vi "NewKickTo.vi"(0 "KickToSkill in":refnum<class "KickToSkill.lvclass">, 1 "Robot":refnum<class "Robot.lvclass">, 2 "State in":T1=enum."walk", 3 "use criteria?":bool, 4 "Game":refnum<class "Game.lvclass">, 5 "error in (no error)":errorcluster, 6 "firstCall?":bool=TRUE, 9 "Target":dbl[](array[numeric]), 13 "pass?":bool, 17 "chipKick ?":bool, 18 "ForceInGame":bool) -> (14 "KickToSkill out":refnum<class "KickToSkill.lvclass">, 15 "Robot out":refnum<class "Robot.lvclass">, 16 "State out":T1=enum."walk", 19 "error out":errorcluster)   [LabVIEW 2020, in "KickToSkill.lvclass"]
uses:
  KickToSkill.lvclass
  Robot_class/Robot.lvclass
  C:/Users/anton/Desktop/RoboIME/SSL_COMP/SSL_AI/Object_class/Object.lvclass
  Game_class/Game.lvclass
  Utilities_class/Utilities.lvclass
  Robot_class/robotKickToStates.ctl
  Robot_class/roles.ctl
  Team_class/OffensivePlay.ctl
  Robot_class/Robot.lvclass/Robot.ctl
  Game_class/Game.lvclass/Game.ctl
  Team_class/Team.lvclass/Team.ctl
  Object_class/Object.lvclass/Object.ctl
  Parameters_class/Parameters.lvclass/Parameters.ctl
  RobotFeedback/RobotFeedback.lvclass/RobotFeedback.ctl
  Robot_class/Write dest_x.vi
  Robot_class/Write dest_y.vi
  Robot_class/Write dest_orientation.vi
  Robot_class/Write dribble.vi
  RobotFeedback/Read dribblerContactToBall.vi
  <vilib>/Analysis/coordinate.llb/Wrap Angle (scalar).vi
  Robot_class/Read dest_orientation.vi
  Robot_class/Read orientation.vi
  Game_class/Read EnemyRef.vi
  Game_class/Read NewParameters.vi
  Game_class/Read FieldRef.vi
  Team_class/Read RobotRef.vi
  <vilib>/Analysis/_algsub.llb/Real Vector Norm.vi
  Object_class/Read x.vi
  Object_class/Read y.vi
  Robot_class/Write kick_x.vi
  Robot_class/Write kick_z.vi
  Parameters_class/Read ShootOutForce.vi
  Parameters_class/Read AttakingOurselves.vi
  Parameters_class/Read DistanceStop.vi
  Object_class/Read position(x,y).vi
  Game_class/Read BallRef.vi
  Game_class/Read Parameters.lvclass.vi
  Game_class/Read Utilities.lvclass.vi
  Game_class/Read OffensiveTeam.vi
  Game_class/Read Referee.vi
  Game_class/Read RobotsFeedback.vi
  Team_class/Read OffensivePlay.vi
  Parameters_class/Read timeoutToShoot.vi
  Parameters_class/Read ForceInGame.vi
  Parameters_class/Read Force++.vi
  Parameters_class/Read ChipKick activated.vi
  Parameters_class/Read KickEps.vi
  Parameters_class/Read KickRange.vi
  Parameters_class/Read MinDistToKick.vi
  Parameters_class/Read DistanceToKickingAngle.vi
  Parameters_class/Read KickAngle.vi
  Parameters_class/Read Enviroment.vi
  Parameters_class/Read KickForce.vi
  Parameters_class/Read TouchDistance.vi
  Parameters_class/Read Shoot Out_.vi
  Parameters_class/Read DistanceToConsiderRobotArrive.vi
  Robot_class/Read id.vi
  Robot_class/Write dest_x_kick.vi
  Robot_class/Write dest_y_kick.vi
  Robot_class/Read role.vi
  Robot_class/Write robotKickState.vi
  Enemy_class/Enemy.lvclass
  C:/Users/anton/Desktop/RoboIME/SSL_COMP/SSL_AI/Team_class/Team.lvclass
  Ally_class/Ally.lvclass
  Ball_class/Ball.lvclass
  Parameters_class/Read AttackerAngleToShootInDegrees.vi
  Parameters_class/Read AttackerAngleToTurnInDegrees.vi
  Field_class/Field.lvclass
  Parameters_class/Parameters.lvclass
  Referee_class/Referee.lvclass
  RobotFeedback/RobotFeedback.lvclass
  <vilib>/Analysis/NI_AAL_Angle.lvlib
  <vilib>/Analysis/NI_AALPro.lvlib
panel:
  out "difAngleRobotBall 4":dbl
  out "difAngleRobotBall 3":dbl
  out "firstCallArray":bool[](array[boolean])
  in  "AttackingOurselves":bool=TRUE
  out "?":refnum<class "Utilities.lvclass">
  out "difAngleRobotBall 2":dbl
  out "difAngleRobotBall":dbl
  out "difInDegrees":dbl
  out "orientationInDegrees":dbl
  out "?":refnum<class "Utilities.lvclass">
  out "?":refnum<class "Utilities.lvclass">
  in  "?":refnum<class "Utilities.lvclass">
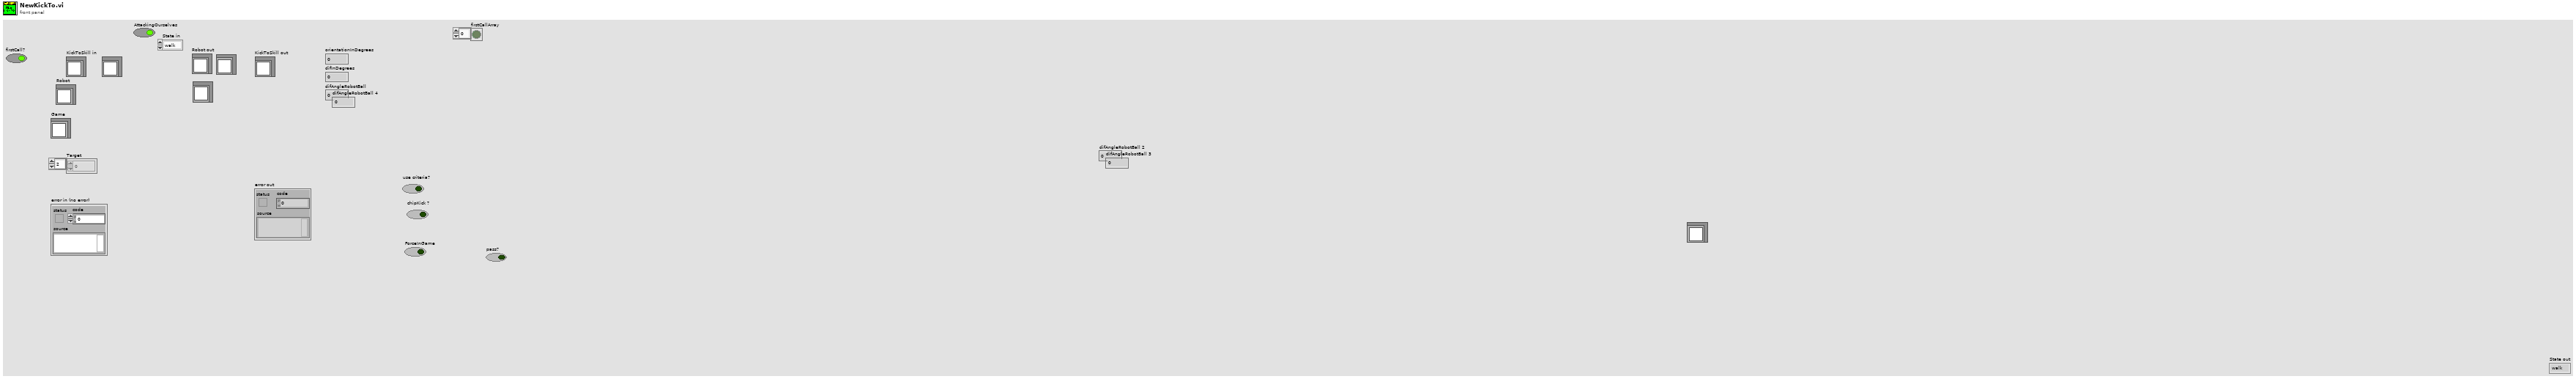
[diagram p1: front panel]
types:
  T1 = typedef "robotKickToStates.ctl" = enum16{"shootFromDirect", "avoidCollideBall", "goToBackBall", "none", "walk", "turn", "oldKickToShoot", "oldKickToGoToBackBall", "shoot"}
  T2 = typedef "OffensivePlay.ctl" = enum16{"5RobotsPassGamePlay", "5PreparePassGame", "5RobotsKeeperGame", "KeeperPassToStriker", "5RobotsNormalGamePlay", "PrepareKeeperPass", "ACBPass", "ABCPass", "PrepareTriplePass", "TableWithStriker", "TableWith2ndStrikerPlay", "PrepareDoublePass", "PrepareRollToPass", "SimplePass", "PreparePass", "PassToStriker", "BallOutOfField", "PassTo2ndStriker", "StopOffensive", "Prepare Penalty Enemy", "EnemyPossessionAtEnemyField", "EnemyPossesionAtOurField", "TestPlay", "PreparePenaltyAlly", "KickPenaltyAlly", "PrepareKickoffAlly", "PrepareKickoffEnemy", "IndirectEnemy", "DirectEnemy", "PreparePassInGame1", "NormalGame", "DirectKick", "Pass", "Halt", "Timeout", "PassPlay", "PenaltyEnemy"}
  T3 = typedef "roles.ctl" = enum16{"SimpleBallPlacement", "BallPlacementAllyPasser", "BallPlacementAllyReceiver", "BallPlacementEnemy", "5Robots5th", "PassBestReceiver", "5Robots4th", "5Robots3rd", "5Robots2nd", "5Robots1st", "PassBestRobot", "WaitPass", "ABCThirdKicker", "ABCFirstKicker", "ABCSecondKicker", "Tabler", "TableFinalizer", "PrepareRollToPassRoller", "PrepareRollToPassReceiver", "SimplePassRoll", "SimplePassRollReceiver", "PenaltyDefense", "PreparePassReceiver 2", "PreparePassReceiver 1", "PassObserver", "Timeout", "Goto", "ZigZag", "None", "BallOutOfField", "DefenderArea", "Duelist", "AttackerStop", "FollowAttacker", "KeeperRole", "KickPenalty", "AttackerAimGoal", "AttackerBlock", "Marker", "Halt", "Shoot", "PassKicker", "PassReceiver", "TestRole", "PenaltyAttacker"}
  T4 = typedef "NewParameters.ctl" = cluster{"PenaltyDistance":dbl, "DistanceAttackerToBackBall":dbl, "Division":enum16{"Div B", "Div A"}, "DistanceToAvoidyEnemyRobot":dbl, "BallPlacementDistance":dbl, "DisatanceBehindBallToStealBall":dbl, "MaxDistanceToPositionKickoff":dbl, "BlockEnemyTarget":bool, "MaxStopVAng":dbl, "DistanceMarkerToEnemy":dbl, "IgnoreDribblerContact":bool, "DistanceToBeginEnemyPosession":dbl, "GoToBallWhenEnemyNotMoving":bool, "EnemyDistanceToReduceVelocity":dbl, "TurnOnEnemyDistanceToReduceVelocity":bool, "EnemyDistanceToShootOutBall":dbl, "DefenseKickBall":bool, "MoreKickToGoal? (0-0.3)":dbl, "ChipKickInEnemyField":bool, "ShootOutRobotId":dbl, "FieldLenghtDenominatorInShootOut":dbl, "AdjustPositionInBallPlacement":bool, "PowerGodPass":dbl, "VelocityAbortEnemyPos":dbl, "MaxDistToBeginPass":dbl, "MinDistToBeginPass":dbl, "VelocityInDirects":dbl, "BadDribblerIDs":i32[], "NewKickToDistanceAroundBall":dbl, "PowerAvoidColisionMarker":dbl, "DistanceToAvoidColisionMarker":dbl, "AvoidBallKick":dbl, "DistanceTryKick":dbl, "SuicideKickDIstance":dbl, "FirstKickAtck":bool, "AdjustFirstKickDistance":dbl, "FirstKickDefense":bool, "AvoidAimLessKick":dbl, "DistanceToAvoidyEnemyShootRobot ":dbl, "NumberOfMarkers":dbl, "PotField":bool, "PIDLateral":bool, "MinDistanceFirstKickX":dbl, "MinDistanceFirstKickY":dbl, "FractionOfDistToTouchGround\nAfterChipKick":dbl, "FractionOfKickxWhen\nComposedWithKickz":dbl, "Style":T5, "MoveInTurnState":bool}
  T5 = typedef "Style.ctl" = enum16{"Insanity", "Offensive", "Defensive"}
  T6 = typedef "Enviroment.ctl" = enum16{"erForceSimulator", "grSim", "realGame"}
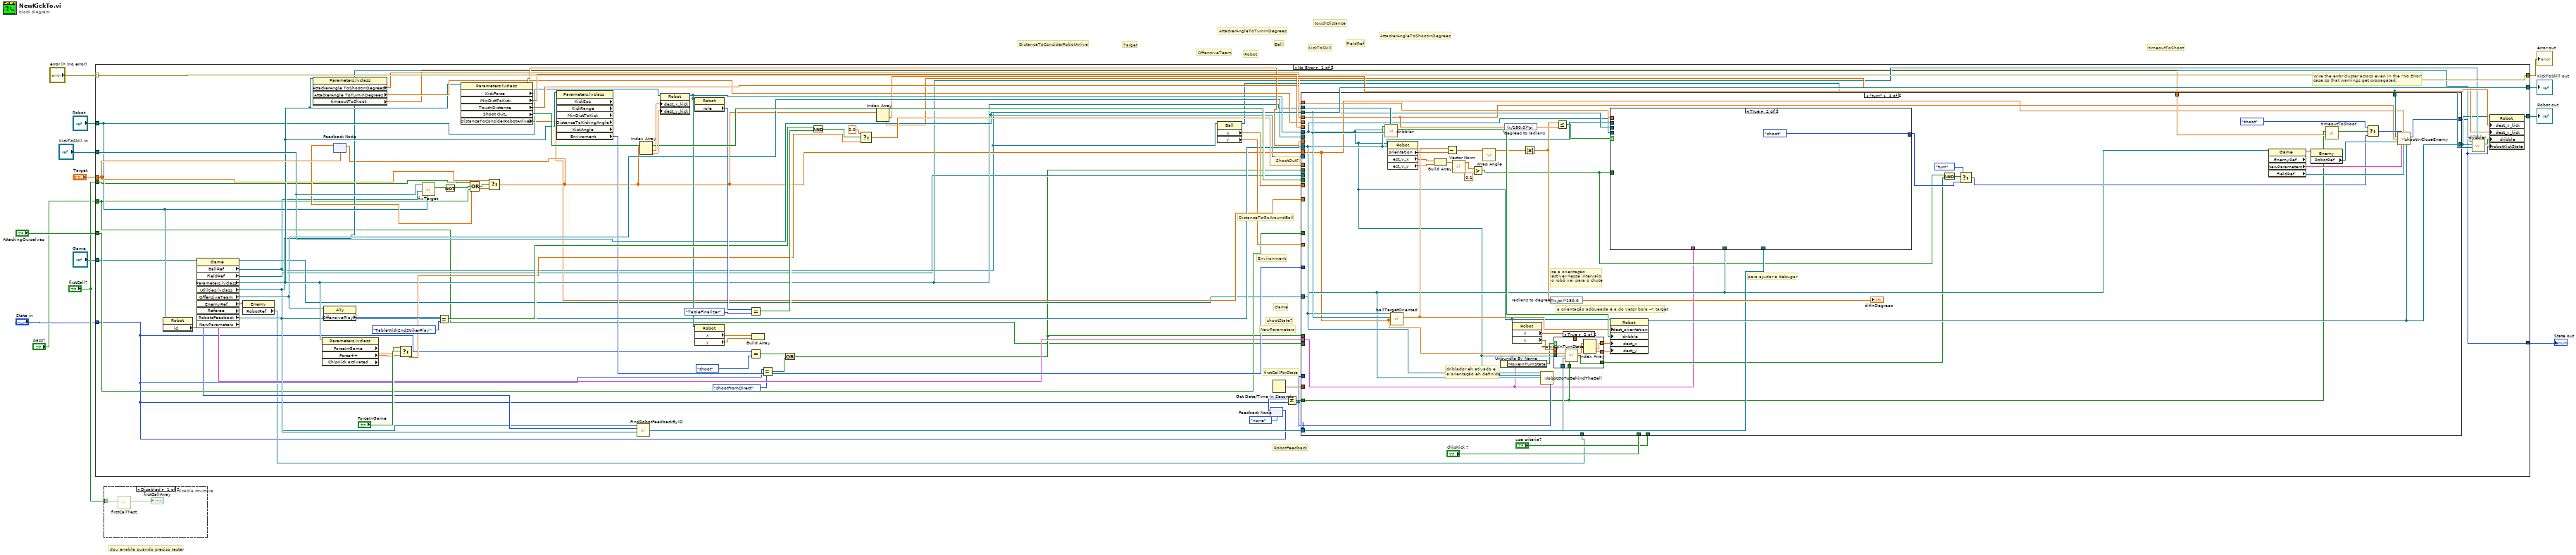
[diagram p0: block diagram]
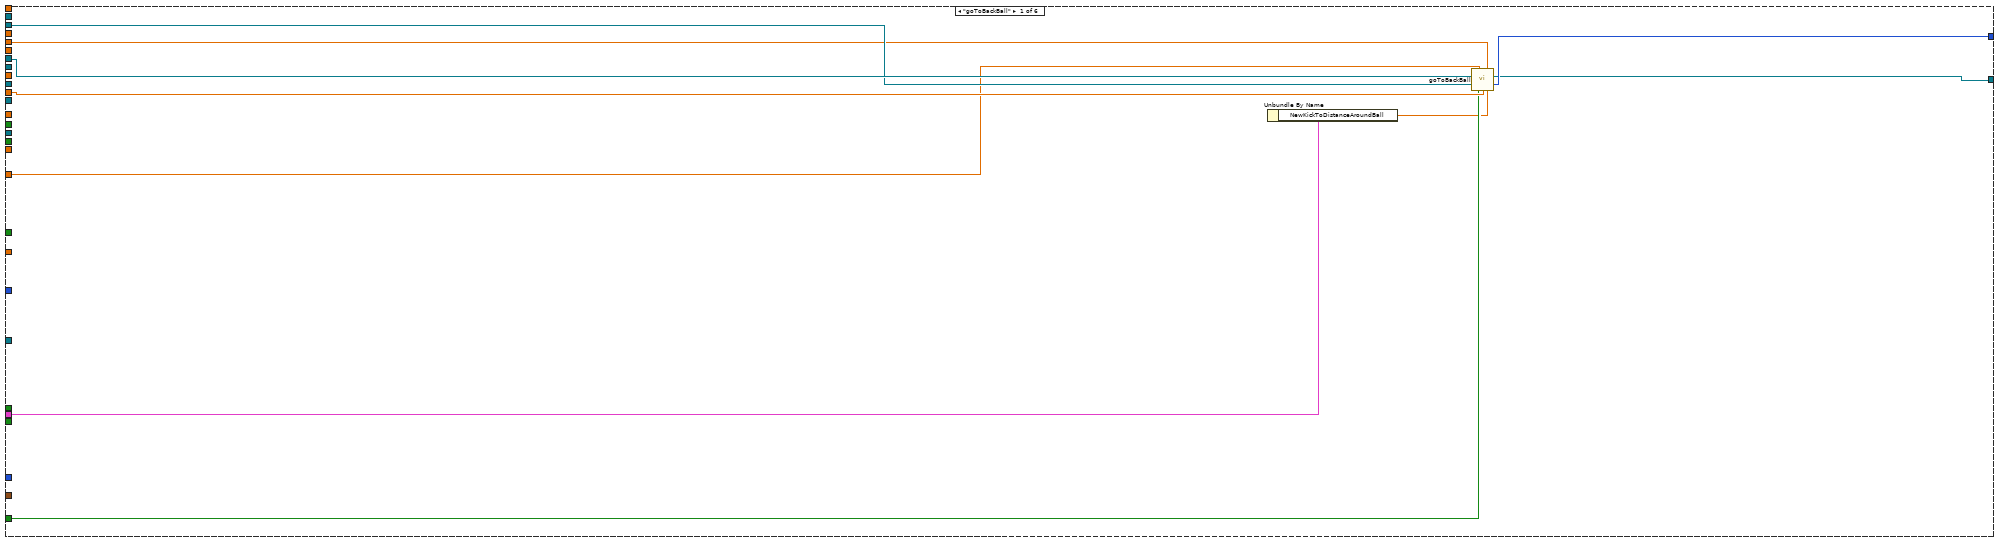
[diagram p2: hidden frame]
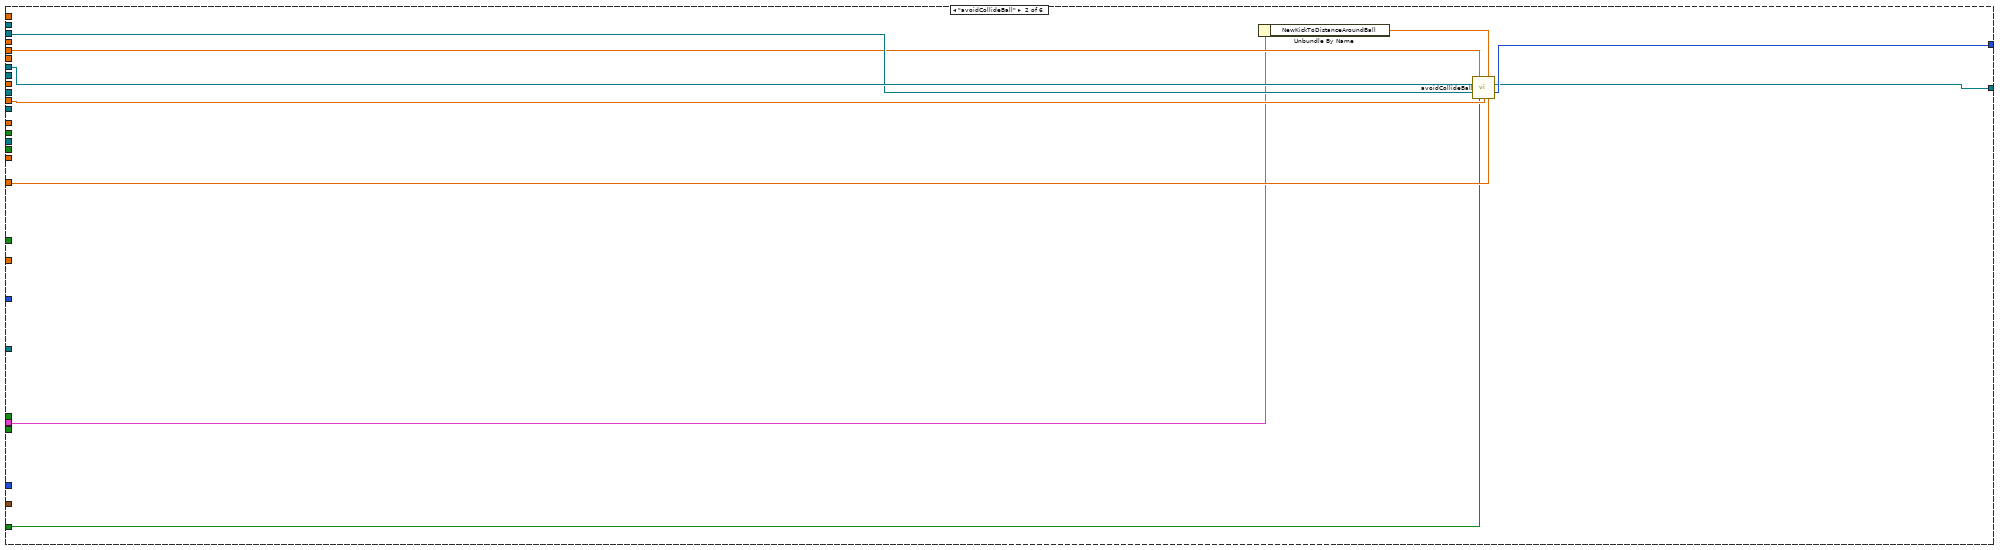
[diagram p3: hidden frame]
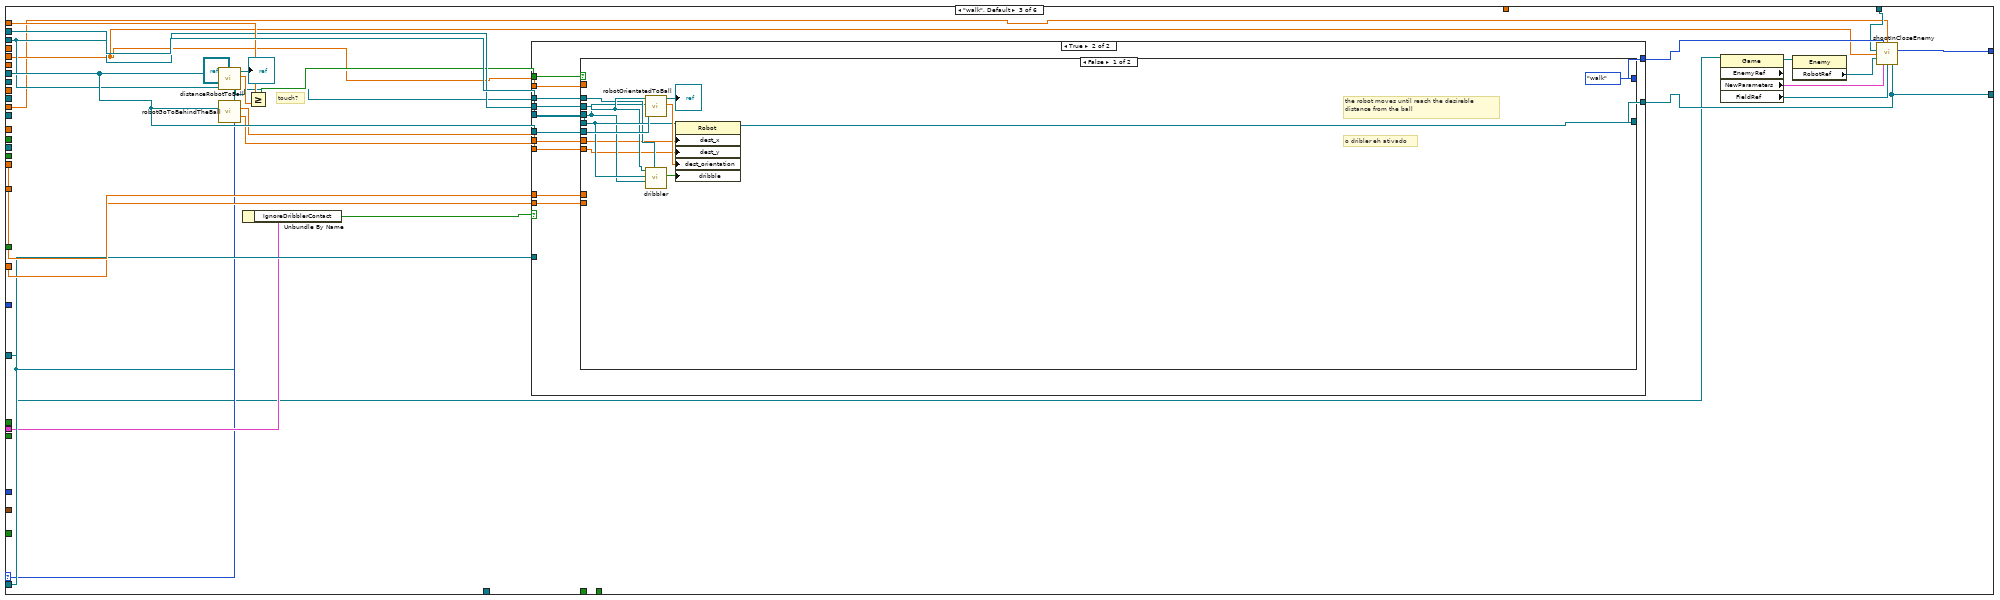
[diagram p4: hidden frame]
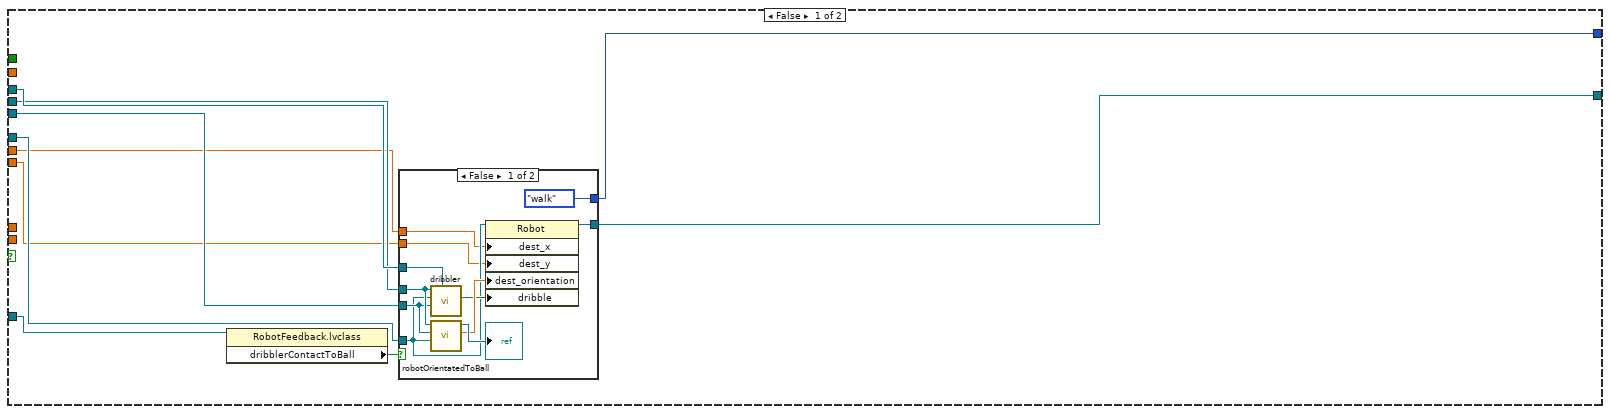
[diagram p5: hidden frame]
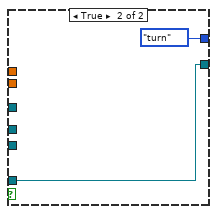
[diagram p6: hidden frame]
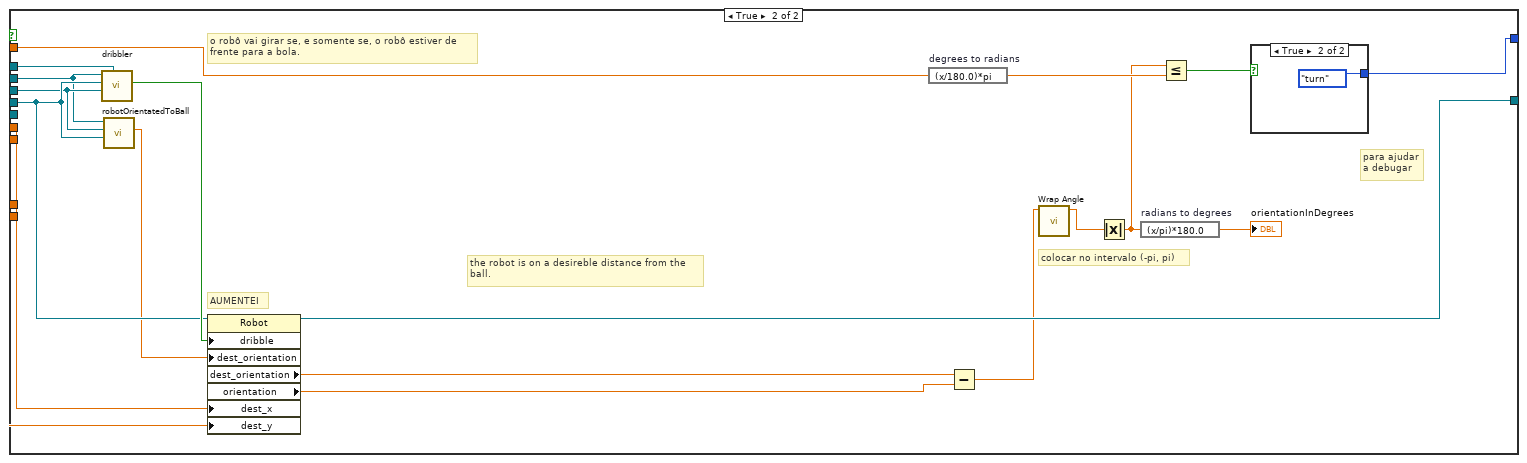
[diagram p7: hidden frame]
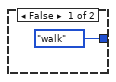
[diagram p8: hidden frame]
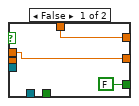
[diagram p9: hidden frame]
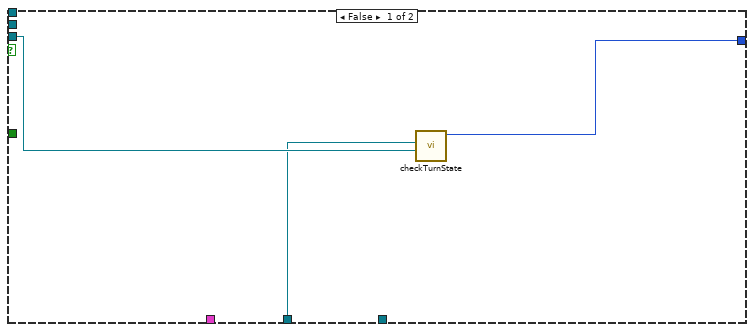
[diagram p10: hidden frame]
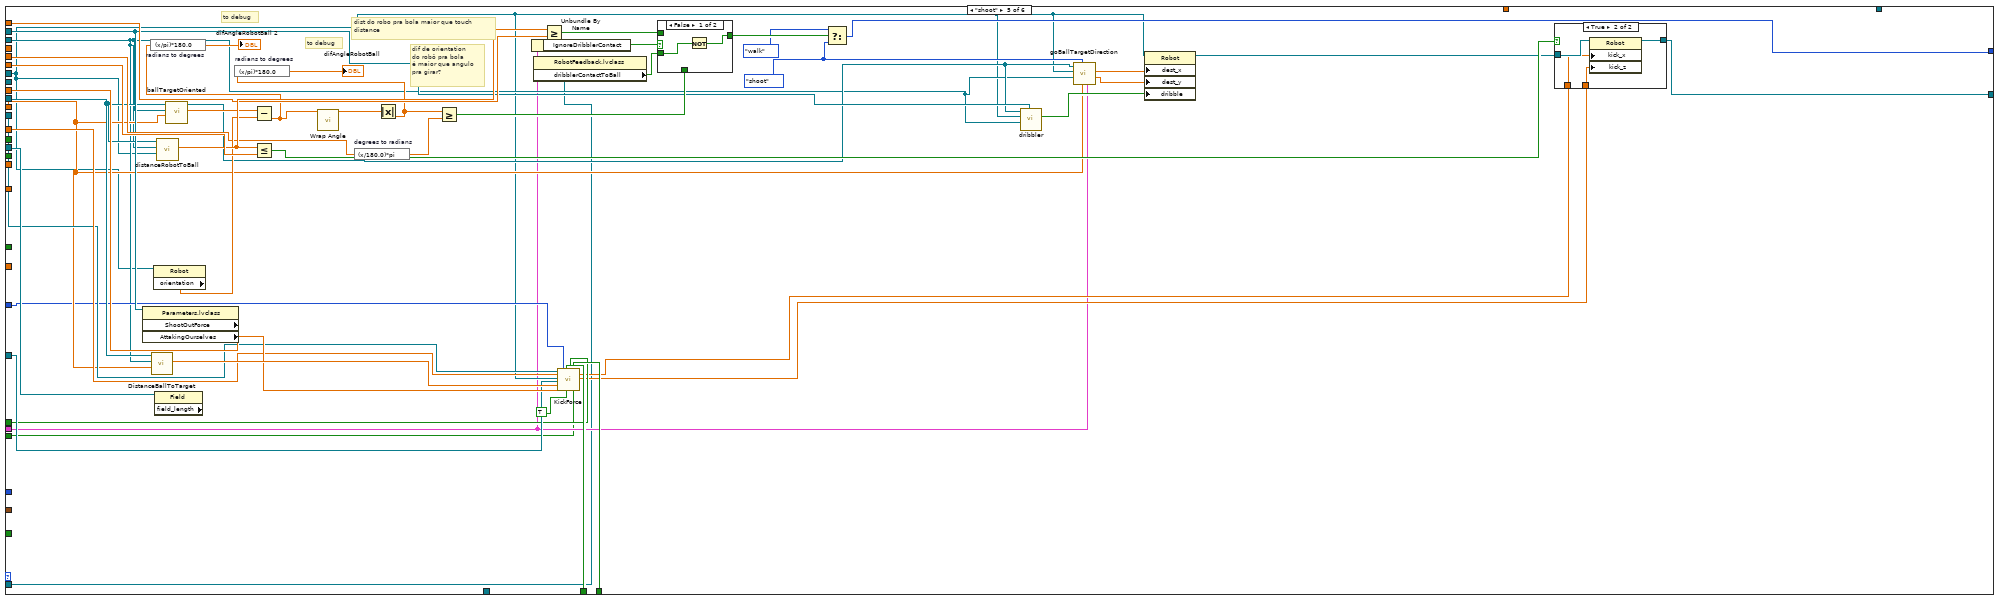
[diagram p11: hidden frame]
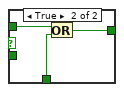
[diagram p12: hidden frame]
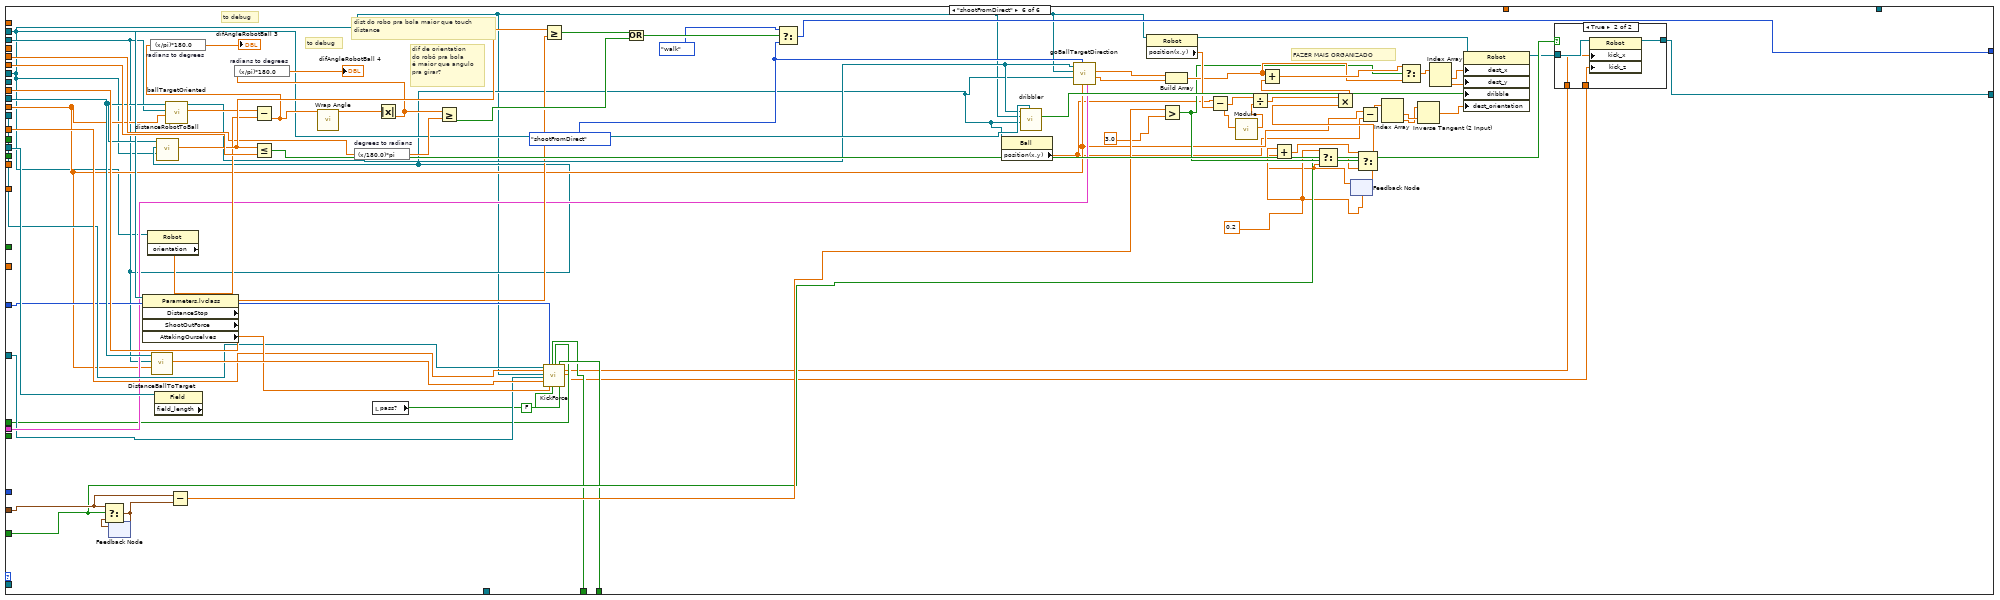
[diagram p14: hidden frame]
diagram:
  # "dou enable quando preciso testar"
  # "timeoutToShoot"
  # "AttackerAngleToShootInDegrees"
  # "touchDistance"
  # "AttackerAngleToTurnInDegrees"
  # "DistanceToConsiderRobotArrive"
  # "FieldRef"
  # "KickToSkill"
  # "Target"
  # "OffensiveTeam"
  # "Robot"
  # "Ball"
  n1 = case shown="No Error" "error in (no error)" {
    selector: "error in (no error)" -> [w86 w402]
    tunnel: [w86 w402] -> w12
    tunnel: [w61 w401] -> w10
    tunnel: "KickToSkill in" -> [w61 w401]
    tunnel: "Robot" -> [w49 w400]
    tunnel: [w57 w400] -> w8
    tunnel: "Game" -> [w27 _]
    tunnel: "Target" -> [w59 _]
    tunnel: "firstCall?" -> [w19 _]
    tunnel: "AttackingOurselves" -> [w43 _]
    tunnel: "State in" -> [w26 _]
    tunnel: [w25 _] -> w2
    tunnel: "pass?" -> [w16 _]
    frame No Error {
      # "RobotFeedback"
      # "shootState?"
      # "Game"
      # "NewParameters"
      # "firstCallForState"
      # "DistanceToGoAroundBall"
      # "Environment"
      # "ShootOut?"
      # "Wire the error cluster across even in the \"No Error\"\ncase so that warnings get propagated."
      n2 = property class="Robot"(reference=w49) -> ("id"=w48:i32)  [unwired: 1 in, 2 out]
      n3 = property class="Game" props=["BallRef", "FieldRef", "Parameters.lvclass", "Utilities.lvclass", "OffensiveTeam", "EnemyRef", "Referee", "RobotsFeedback", "NewParameters"](reference=w27) -> (reference out=w33:refnum<class "Game.lvclass">, "BallRef"=w32:refnum<class "Ball.lvclass">, "FieldRef"=w31:refnum<class "Field.lvclass">, "Parameters.lvclass"=w51:refnum<class "Parameters.lvclass">, "Utilities.lvclass"=w46:refnum<class "Utilities.lvclass">, "OffensiveTeam"=w60:refnum<class "Ally.lvclass">, "EnemyRef"=w15:refnum<class "Enemy.lvclass">, "RobotsFeedback"=w47:refnum<class "RobotFeedback.lvclass">[], "NewParameters"=w36:T4)  [unwired: 1 in, 2 out]
      n4 = property class="Enemy"(reference=w15) -> ("RobotRef"=w14:refnum<class "Robot.lvclass">[])  [unwired: 1 in, 2 out]
      n5 = property class="Parameters.lvclass"(reference=w51) -> ("AttackerAngle ToShootInDegrees"=w53:dbl, "AttackerAngle ToTurnInDegrees"=w54:dbl, "timeoutToShoot"=w37:dbl)  [unwired: 1 in, 2 out]
      n6 = property class="Parameters.lvclass" props=["ForceInGame", "Force++", "ChipKick activated"](reference=w51) -> ("ForceInGame"=w68:dbl, "Force++"=w67:dbl)  [unwired: 1 in, 3 out]
      n7 = property class="Ally"(reference=w60) -> ("OffensivePlay"=w73:T2)  [unwired: 1 in, 2 out]
      n8 = feedback #1(w59) -> (w58:dbl[])
      n9 = Select(t=w68, s="ForceInGame", f=w67) -> (s? t:f=w66:dbl)
      n10 = call "fixTarget.vi"("Robot"=w49, "Ball"=w32, "KickToSkill in"=w61) -> ("fixTarget?"=w24:bool)  [unwired: 6 in, 2 out]
      n11 = Equal?(x=w73, y=OffensivePlay."TableWith2ndStrikerPlay") -> (x = y?=w71:bool)
      n12 = Not(x=w24) -> (.not. x?=w18:bool)
      n13 = property class="Parameters.lvclass"(reference=w51) -> ("KickForce"=w78:dbl, "MinDistToKick"=w85:dbl, "TouchDistance"=w84:dbl, "Shoot Out_"=w79:bool, "DistanceToConsiderRobotArrive"=w41:dbl)  [unwired: 1 in, 2 out]
      n14 = Compound Arithmetic op=OR(w19, w18, w16) -> (w17:bool)
      n15 = Select(t=w59, s=w17, f=w58) -> (s? t:f=w42:dbl[])
      n16 = feedback-in #1(w42) -> ()
      n17 = property class="Parameters.lvclass" props=["KickEps", "KickRange", "MinDistToKick", "DistanceToKickingAngle", "KickAngle", "Enviroment"](reference=w51) -> ("Enviroment"=w45:T6)  [unwired: 1 in, 7 out]
      n18 = call "FindRobotFeedbackByID.vi"("RobotsFeedback"=w47, "id"=w48, "Utilities in"=w46) -> ("RobotFeedback.lvclass"=w44:refnum<class "RobotFeedback.lvclass">)  [unwired: 5 in, 3 out]
      n19 = Index Array(array=w42) -> (element #1=w81:dbl, element #2=w80:dbl)  [unwired: 2 in]
      n20 = property class="Robot"(reference=w49, "dest_x_kick"=w81, "dest_y_kick"=w80) -> (reference out=w62:refnum<class "Robot.lvclass">)  [unwired: 1 in, 1 out]
      n21 = property class="Robot"(reference=w62) -> ("role"=w76:T3)  [unwired: 1 in, 2 out]
      n22 = property class="Robot"(reference=w62) -> ("x"=w65:dbl, "y"=w64:dbl)  [unwired: 1 in, 2 out]
      n23 = Equal?(x=w76, y=roles."TableFinalizer") -> (x = y?=w74:bool)
      n24 = Equal?(x=w26, y=robotKickToStates."shoot" ("robotKickState")) -> (x = y?=w30:bool)
      n25 = Build Array(w65, w64) -> ()  [unwired: 1 out]
      n26 = Equal?(x=w26, y=robotKickToStates."shootFromDirect") -> (x = y?=w29:bool)
      n27 = Or(x=w30, y=w29) -> (x .or. y?=w20:bool)
      n28 = And(x=w71, y=w74) -> (x .and. y?=w70:bool)
      n29 = Select(t=0.0, s=w70, f=w66) -> (s? t:f=w63:dbl)
      n30 = Index Array(array=w42) -> (element #1=w56:dbl, element #2=w55:dbl)  [unwired: 2 in]
      n31 = property class="Ball"(reference=w32) -> (reference out=w34:refnum<class "Ball.lvclass">, "x"=w82:dbl, "y"=w83:dbl)  [unwired: 1 in, 1 out]
      n32 = feedback #2(robotKickToStates."none" ("state out")) -> (w40:T1)
      n33 = feedback-in #2(w26) -> ()
      n34 = Get Date/Time In Seconds() -> (seconds since 1Jan1904=w35:timestamp)
      n35 = Not Equal?(x=w40, y=w26) -> (x != y?=w39:bool)
      n36 = case shown="\"turn\"" w26 {
        selector: w26 -> [_ _ w109 w225 _ _]
        tunnel: [w96 w106 w119 w235 w295 w378] -> w25
        tunnel: w82 -> [_ _ w133 _ _ _]
        tunnel: w83 -> [_ _ w132 _ _ _]
        tunnel: w62 -> [w94 w104 w129 w222 w277 w330]
        tunnel: [w95 w105 w112 w229 w310 w392] -> w50
        tunnel: w32 -> [w93 w103 w128 w241 w279 w332]
        tunnel: w51 -> [_ _ w131 w250 w286 w369]
        tunnel: w84 -> [_ _ w130 w246 w302 _]
        tunnel: w46 -> [_ _ _ w240 w285 w368]
        tunnel: w85 -> [_ _ _ _ w312 w394]
        tunnel: w78 -> [_ _ _ _ w307 w389]
        tunnel: w61 -> [_ _ _ _ w305 w387]
        tunnel: w60 -> [_ _ _ _ _ _]
        tunnel: w31 -> [_ _ _ _ w308 w390]
        tunnel: w79 -> [_ _ _ _ _ _]
        tunnel: w42 -> [w92 w102 w108 w223 w284 w338]
        tunnel: w63 -> [_ _ _ _ w306 w388]
        tunnel: w20 -> [_ _ _ _ _ _]
        tunnel: w54 -> [w90 w100 w111 _ w293 w376]
        tunnel: w53 -> [_ _ _ w228 _ _]
        tunnel: w26 -> [_ _ _ _ _ _]
        tunnel: w45 -> [_ _ _ _ w281 w367]
        tunnel: w44 -> [_ _ w121 w226 w269 _]
        tunnel: w43 -> [_ _ _ _ _ _]
        tunnel: w41 -> [w91 w101 _ _ _ _]
        tunnel: w39 -> [w89 w99 _ w220 _ w343]
        tunnel: w37 -> [_ _ _ w237 _ _]
        tunnel: w36 -> [w88 w98 w120 w203 w270 w364]
        tunnel: w35 -> [_ _ _ _ _ w362]
        tunnel: w34 -> [_ _ w117 w234 _ _]
        tunnel: w33 -> [_ _ w107 w224 w278 w331]
        tunnel: "chipKick ?" -> [_ _ _ _ w276 w327]
        tunnel: "use criteria?" -> [_ _ _ _ w275 w329]
        tunnel: w20 -> [_ _ _ _ w274 w328]
        tunnel: w16 -> [_ _ _ _ w266 _]
        tunnel: w14 -> [_ _ _ w221 _ _]
        frame "goToBackBall" {
          n37 = Unbundle By Name(w88) -> ("NewKickToDistanceAroundBall"=w87:dbl)
          n38 = call "goToBackBall.vi"("DistanceToConsiderRobotArrive"=w91, "AttackerAngle\nToTurnInDegrees"=w90, "Robot in"=w94, "Ball"=w93, "firstCallForState"=w89, "target"=w92, "DistanceToGoAroundBall"=w87) -> ("Robot out"=w95:refnum<class "Robot.lvclass">, "robotKickState"=w96:T1)  [unwired: 5 in, 2 out]
        }
        frame "avoidCollideBall" {
          n39 = Unbundle By Name(w98) -> ("NewKickToDistanceAroundBall"=w97:dbl)
          n40 = call "avoidCollideBall.vi"("AttackerAngle\nToTurnInDegrees"=w100, "DistanceToGoAroundBall"=w97, "Robot"=w104, "Ball"=w103, "firstCallForState"=w99, "Target"=w102, "DistanceToConsiderRobotArrive"=w101) -> ("Robot out"=w105:refnum<class "Robot.lvclass">, "robotKickState"=w106:T1)  [unwired: 5 in, 2 out]
        }
        frame "walk", Default {
          # "touch?"
          n41 = call "distanceRobotToBall.vi"("Robot"=w129, "Ball"=w128, "Utilities in"="?") -> ("Distance Robot To Ball"=w127:dbl, "Utilities out"=→"?":refnum<class "Utilities.lvclass">)  [unwired: 6 in, 1 out]
          n42 = call "robotGoToBehindTheBall.vi"("Utilities in"="?", "Robot"=w129, "Game"=w107, "State in"=w109) -> ("dest_x"=w124:dbl, "dest_y"=w123:dbl)  [unwired: 8 in, 2 out]
          n43 = Unbundle By Name(w120) -> ("IgnoreDribblerContact"=w110:bool)
          n44 = Greater Or Equal?(x=w130, y=w127) -> (x >= y?=w126:bool)
          n45 = case shown="True" w110 {
            tunnel: [w137 w168] -> w118
            tunnel: w133 -> [_ w167]
            tunnel: w132 -> [_ w166]
            tunnel: [w138 w165] -> w112
            tunnel: w131 -> [w142 w164]
            tunnel: w129 -> [w140 w163]
            tunnel: w128 -> [w136 w162]
            tunnel: w111 -> [_ w161]
            tunnel: w126 -> [_ w160]
            tunnel: w124 -> [w135 w159]
            tunnel: w123 -> [w134 w158]
            tunnel: "?" -> [w141 w157]
            tunnel: w121 -> [w143 _]
            frame False {
              n46 = property class="RobotFeedback.lvclass"(reference=w143) -> ("dribblerContactToBall"=w139:bool)  [unwired: 1 in, 2 out]
              n47 = case shown="False" w139 {
                tunnel: w142 -> [w151 _]
                tunnel: w141 -> [w150 _]
                tunnel: w136 -> [w149 _]
                tunnel: w140 -> [w148 w156]
                tunnel: [w147 w156] -> w138
                tunnel: [robotKickToStates."walk" robotKickToStates."turn" ("robotKickState")] -> w137
                tunnel: w135 -> [w145 _]
                tunnel: w134 -> [w144 _]
                frame False {
                  n48 = call "dribbler.vi"("Parameters.lvclass"=w151, "Ball"=w149, "Robot"=w148, "Utilities in"=w150) -> ("Dribbler?"=w152:bool)  [unwired: 5 in, 2 out]
                  n49 = call "robotOrientatedToBall.vi"("Robot"=w148, "BallRef"=w149, "Utilities in"=w150) -> ("Orientation"=w153:dbl, "Utilities out"=→"?":refnum<class "Utilities.lvclass">)  [unwired: 6 in, 1 out]
                  n50 = property class="Robot"(reference=w148, "dest_x"=w145, "dest_y"=w144, "dest_orientation"=w153, "dribble"=w152) -> (reference out=w147:refnum<class "Robot.lvclass">)  [unwired: 1 in, 1 out]
                }
                frame True {
                }
              }
            }
            frame True {
              n51 = case shown="False" w160 {
                tunnel: [robotKickToStates."walk" w198] -> w168
                tunnel: w167 -> [_ _]
                tunnel: w166 -> [_ _]
                tunnel: w163 -> [w176 w195]
                tunnel: [w180 w197] -> w165
                tunnel: w163 -> [w179 _]
                tunnel: w162 -> [w173 w194]
                tunnel: w157 -> [w175 w193]
                tunnel: w164 -> [w174 w199]
                tunnel: w159 -> [w171 w183]
                tunnel: w158 -> [w170 w182]
                tunnel: w161 -> [_ w181]
                frame False {
                  # "o dribler eh ativado"
                  # "the robot moves until reach the desireble \ndistance from the ball"
                  n52 = call "robotOrientatedToBall.vi"("Robot"=w179, "BallRef"=w173, "Utilities in"=w175) -> ("Orientation"=w177:dbl, "Utilities out"=→"?":refnum<class "Utilities.lvclass">)  [unwired: 6 in, 1 out]
                  n53 = call "dribbler.vi"("Parameters.lvclass"=w174, "Ball"=w173, "Robot"=w176, "Utilities in"=w175) -> ("Dribbler?"=w172:bool)  [unwired: 5 in, 2 out]
                  n54 = property class="Robot"(reference=w176, "dest_x"=w171, "dest_y"=w170, "dest_orientation"=w177, "dribble"=w172) -> (reference out=w180:refnum<class "Robot.lvclass">)  [unwired: 1 in, 1 out]
                }
                frame True {
                  # "para ajudar\na debugar"
                  # "colocar no intervalo (-pi, pi)"
                  # "AUMENTEI"
                  # "o robô vai girar se, e somente se, o robô estiver de frente para a bola."
                  # "the robot is on a desireble distance from the\nball."
                  n55 = call "dribbler.vi"("Parameters.lvclass"=w199, "Ball"=w194, "Robot"=w195, "Utilities in"=w193) -> ("Dribbler?"=w196:bool)  [unwired: 5 in, 2 out]
                  n56 = call "robotOrientatedToBall.vi"("Robot"=w195, "BallRef"=w194, "Utilities in"=w193) -> ("Orientation"=w192:dbl)  [unwired: 6 in, 2 out]
                  n57 = property class="Robot"(reference=w195, "dribble"=w196, "dest_orientation"=w192, "dest_x"=w183, "dest_y"=w182) -> (reference out=w197:refnum<class "Robot.lvclass">, "dest_orientation"=w190:dbl, "orientation"=w189:dbl)  [unwired: 1 in, 1 out]
                  n58 = expression code="(x/180.0)*pi" "degrees to radians"(w181) -> (w191:dbl)
                  n59 = Subtract(x=w190, y=w189) -> (x-y=w187:dbl)
                  n60 = call-poly <vilib>:"Wrap Angle.vi"("angle in"=w187) -> ("angle out"=w186:dbl)  [unwired: 9 in, 1 out]
                  n61 = Absolute Value(x=w186) -> (abs(x)=w184:dbl)
                  n62 = expression code="(x/pi)*180.0" "radians to degrees"(w184) -> (→"orientationInDegrees":dbl)
                  n63 = Less Or Equal?(x=w184, y=w191) -> (x <= y?=w188:bool)
                  n64 = case shown="True" w188 {
                    tunnel: [robotKickToStates."walk" robotKickToStates."turn" ("robotKickState")] -> w198
                    frame False {
                    }
                    frame True {
                    }
                  }
                }
              }
            }
          }
          n65 = property class="Game"(reference=w107) -> ("EnemyRef"=w116:refnum<class "Enemy.lvclass">, "NewParameters"=w114:T4, "FieldRef"=w113:refnum<class "Field.lvclass">)  [unwired: 1 in, 2 out]
          n66 = property class="Enemy"(reference=w116) -> ("RobotRef"=w115:refnum<class "Robot.lvclass">[])  [unwired: 1 in, 2 out]
          n67 = call "shootInCloseEnemy.vi"("robotKickState In"=w118, "Target"=w108, "Ball"=w117, "AttackerAngle ToShootInDegrees"=w111, "EnemyRoboRef"=w115, "NewParameters"=w114, "FieldRef"=w113, "Robot in"=w112) -> ("robotKickState out"=w119:T1)  [unwired: 5 in, 2 out]
        }
        frame "turn" {
          # "para ajudar a debugar"
          # "a orientação adqueada é a do vetor bola -> target"
          # "se a orientação \nestiver nesse intervalo\no robô vai para o chute"
          # "driblador eh ativado e\na orientação eh definida"
          n68 = call "dribbler.vi"("Parameters.lvclass"=w250, "Ball"=w241, "Robot"=w222, "Utilities in"=w240) -> ("Dribbler?"=w247:bool)  [unwired: 5 in, 2 out]
          n69 = property class="Robot"(reference=w222) -> ("orientation"=w249:dbl, "est_v_x"=w216:dbl, "est_v_y"=w215:dbl)  [unwired: 1 in, 2 out]
          n70 = call "ballTargetOriented.vi"("Target"=w223, "Ball"=w241, "Utilities in"=w240) -> ("Orientation"=w239:dbl)  [unwired: 6 in, 2 out]
          n71 = Build Array(w216, w215) -> (w214:dbl[])
          n72 = Subtract(x=w239, y=w249) -> (x-y=w245:dbl)
          n73 = call-poly <vilib>:"Vector Norm.vi"("Input Vector"=w214) -> ("norm"=w213:dbl)  [unwired: 9 in, 1 out]
          n74 = Greater?(x=w213, y=0.1) -> (0:w207:bool)
          n75 = call-poly <vilib>:"Wrap Angle.vi"("angle in"=w245) -> ("angle out"=w244:dbl)  [unwired: 9 in, 1 out]
          n76 = Unbundle By Name(w203) -> ("MoveInTurnState"=w202:bool)
          n77 = expression code="(x/180.0)*pi" "degrees to radians"(w228) -> (w248:dbl)
          n78 = property class="Robot"(reference=w222) -> ("x"=w205:dbl, "y"=w204:dbl)  [unwired: 1 in, 2 out]
          n79 = Absolute Value(x=w244) -> (abs(x)=w243:dbl)
          n80 = call "robotGoToBehindTheBall.vi"("Utilities in"=w240, "Robot"=w222, "Game"=w224, "State in"=w225) -> ()  [unwired: 8 in, 4 out]
          n81 = expression code="(x/pi)*180.0" "radians to degrees"(w243) -> (→"difInDegrees":dbl)
          n82 = case shown="True" w202 {
            tunnel: w223 -> [_ w261]
            tunnel: w222 -> [_ w260]
            tunnel: w221 -> [_ w259]
            tunnel: w220 -> [_ w258]
            tunnel: [w253 w256] -> w219
            tunnel: [w252 w255] -> w218
            tunnel: [FALSE ("RobotToClose") w254] -> w208
            tunnel: w205 -> [w253 _]
            tunnel: w204 -> [w252 _]
            frame False {
            }
            frame True {
              n83 = call "movingInTurnState.vi"("Target"=w261, "Robot"=w260, "RobotRef"=w259, "first call"=w258) -> ("Dest"=w257:dbl[], "RobotToClose"=w254:bool)  [unwired: 8 in, 2 out]
              n84 = Index Array(array=w257) -> (element #1=w256:dbl, element #2=w255:dbl)  [unwired: 2 in]
            }
          }
          n85 = Less Or Equal?(x=w243, y=w248) -> (x <= y?=w217:bool)
          n86 = case shown="True" w217 {
            tunnel: [w262 robotKickToStates."shoot" ("robotKickState")] -> w210
            tunnel: w240 -> [_ _]
            tunnel: w222 -> [w264 _]
            tunnel: w241 -> [_ _]
            tunnel: w246 -> [_ _]
            tunnel: w203 -> [_ _]
            tunnel: w226 -> [_ _]
            tunnel: w224 -> [w263 _]
            tunnel: w207 -> [_ _]
            frame False {
              n87 = call "checkTurnState.vi"("Robot"=w264, "Game"=w263) -> ("robotKickState"=w262:T1)  [unwired: 9 in]
            }
            frame True {
            }
          }
          n88 = property class="Robot"(reference=w222, "dest_orientation"=w239, "dribble"=w247, "dest_x"=w219, "dest_y"=w218) -> (reference out=w229:refnum<class "Robot.lvclass">)  [unwired: 1 in, 1 out]
          n89 = And(x=w207, y=w208) -> (x .and. y?=w206:bool)
          n90 = Select(t=robotKickToStates."turn" ("robotKickState"), s=w206, f=w210) -> (s? t:f=w209:T1)
          n91 = property class="Game"(reference=w224) -> ("EnemyRef"=w233:refnum<class "Enemy.lvclass">, "NewParameters"=w231:T4, "FieldRef"=w230:refnum<class "Field.lvclass">)  [unwired: 1 in, 2 out]
          n92 = property class="Enemy"(reference=w233) -> ("RobotRef"=w232:refnum<class "Robot.lvclass">[])  [unwired: 1 in, 2 out]
          n93 = call "timeoutToShoot.vi"("timeoutToShoot"=w237, "firstCallForState"=w220) -> ("elapsedTimeToShoot"=w238:bool)  [unwired: 7 in, 2 out]
          n94 = Select(t=robotKickToStates."shoot" ("robotKickState"), s=w238, f=w209) -> (s? t:f=w236:T1)
          n95 = call "shootInCloseEnemy.vi"("robotKickState In"=w236, "Target"=w223, "Ball"=w234, "AttackerAngle ToShootInDegrees"=w228, "EnemyRoboRef"=w232, "NewParameters"=w231, "FieldRef"=w230, "Robot in"=w229) -> ("robotKickState out"=w235:T1)  [unwired: 5 in, 2 out]
        }
        frame "shoot" {
          w280 = robotKickToStates."shoot" ("robotKickState")
          # "to debug"
          # "to debug"
          # "dif de orientation\ndo robô pra bola\né maior que angulo\npra girar?"
          # "dist do robo pra bola maior que touch\ndistance"
          n96 = property class="Parameters.lvclass" props=["ShootOutForce", "AttakingOurselves"](reference=w286) -> ()  [unwired: 1 in, 4 out]
          n97 = call-dynamic "DistanceBallToTarget.vi"("Target"=w284, "Ball"=w279, "Utilities in"=w285) -> ("Distance Ball To Target"=w309:dbl)  [unwired: 6 in, 2 out]
          n98 = property class="Robot"(reference=w277) -> ("orientation"=w299:dbl)  [unwired: 1 in, 2 out]
          n99 = property class="Field" props=["field_length"](reference=w308) -> ()  [unwired: 1 in, 3 out]
          n100 = call "distanceRobotToBall.vi"("Robot"=w277, "Ball"=w279, "Utilities in"=w285) -> ("Distance Robot To Ball"=w303:dbl)  [unwired: 6 in, 2 out]
          n101 = call "ballTargetOriented.vi"("Target"=w284, "Ball"=w279) -> ("Orientation"=w300:dbl)  [unwired: 7 in, 2 out]
          n102 = Subtract(x=w300, y=w299) -> (x-y=w289:dbl)
          n103 = expression code="(x/pi)*180.0" "radians to degrees"(w289) -> (→"difAngleRobotBall 2":dbl)
          n104 = Less Or Equal?(x=w303, y=w312) -> (x <= y?=w311:bool)
          n105 = call-poly <vilib>:"Wrap Angle.vi"("angle in"=w289) -> ("angle out"=w301:dbl)  [unwired: 9 in, 1 out]
          n106 = expression code="(x/180.0)*pi" "degrees to radians"(w293) -> (w294:dbl)
          n107 = Absolute Value(x=w301) -> (abs(x)=w292:dbl)
          n108 = expression code="(x/pi)*180.0" "radians to degrees"(w292) -> (→"difAngleRobotBall":dbl)
          n109 = Greater Or Equal?(x=w292, y=w294) -> (x >= y?=w298:bool)
          n110 = Unbundle By Name(w270) -> ("IgnoreDribblerContact"=w268:bool)
          n111 = property class="RobotFeedback.lvclass"(reference=w269) -> ("dribblerContactToBall"=w267:bool)  [unwired: 1 in, 2 out]
          n112 = Greater Or Equal?(x=w303, y=w302) -> (x >= y?=w304:bool)
          n113 = call "KickForce.vi"("KickToSkill in"=w305, "force++"=w306, "Robot"=w277, "Game"=w278, "Distance to target"=w309, "Enviroment"=w281, "kickForce"=w307, "chipKick ?"=w276, "weakKick?"=TRUE, "shootState?"=w274, "use criteria?"=w275, "pass?"=w266) -> ("kick_x Force out"=w273:dbl, "kick_z Force out"=w272:dbl)  [unwired: 4 in, 2 out]
          n114 = case shown="False" w268 {
            tunnel: w304 -> [_ w317]
            tunnel: w298 -> [_ w316]
            tunnel: [w313 w315] -> w297
            tunnel: w267 -> [w314 _]
            frame False {
              n115 = Not(x=w314) -> (.not. x?=w313:bool)
            }
            frame True {
              n116 = Or(x=w317, y=w316) -> (x .or. y?=w315:bool)
            }
          }
          n117 = Select(t=robotKickToStates."walk", s=w297, f=w280) -> (s? t:f=w295:T1)
          n118 = call "dribbler.vi"("Parameters.lvclass"=w286, "Ball"=w279, "Robot"=w277, "Utilities in"=w285) -> ("Dribbler?"=w287:bool)  [unwired: 5 in, 2 out]
          n119 = call-dynamic "goBallTargetDirection.vi"("NewParameters"=w270, "Target"=w284, "state"=w280, "BallRef"=w279, "Robot"=w277, "Utilities in"=w285) -> ("dest_y"=w282:dbl, "dest_x"=w283:dbl)  [unwired: 2 in, 2 out]
          n120 = property class="Robot"(reference=w277, "dest_x"=w283, "dest_y"=w282, "dribble"=w287) -> (reference out=w288:refnum<class "Robot.lvclass">)  [unwired: 1 in, 1 out]
          n121 = case shown="True" w311 {
            tunnel: w288 -> [w318 w322]
            tunnel: [w318 w321] -> w310
            tunnel: w273 -> [_ w320]
            tunnel: w272 -> [_ w319]
            frame False {
            }
            frame True {
              n122 = property class="Robot"(reference=w322, "kick_x"=w320, "kick_z"=w319) -> (reference out=w321:refnum<class "Robot.lvclass">)  [unwired: 1 in, 1 out]
            }
          }
        }
        frame "shootFromDirect" {
          w342 = 0.2 ("y")
          w365 = robotKickToStates."shootFromDirect"
          # "FAZER MAIS ORGANIZADO"
          # "to debug"
          # "to debug"
          # "dif de orientation\ndo robô pra bola\né maior que angulo\npra girar?"
          # "dist do robo pra bola maior que touch\ndistance"
          n123 = feedback #3() -> (w363:timestamp)  [unwired: 1 in]
          n124 = Select(t=w362, s=w343, f=w363) -> (s? t:f=w361:timestamp)
          n125 = feedback-in #3(w361) -> ()
          n126 = property class="Parameters.lvclass" props=["DistanceStop", "ShootOutForce", "AttakingOurselves"](reference=w369) -> ("DistanceStop"=w366:dbl)  [unwired: 1 in, 4 out]
          n127 = property class="Robot"(reference=w330) -> ("orientation"=w382:dbl)  [unwired: 1 in, 2 out]
          n128 = call-dynamic "DistanceBallToTarget.vi"("Target"=w338, "Ball"=w332, "Utilities in"=w368) -> ("Distance Ball To Target"=w391:dbl)  [unwired: 6 in, 2 out]
          n129 = property class="Field" props=["field_length"](reference=w390) -> ()  [unwired: 1 in, 3 out]
          n130 = call "distanceRobotToBall.vi"("Robot"=w330, "Ball"=w332, "Utilities in"=w368) -> ("Distance Robot To Ball"=w385:dbl)  [unwired: 6 in, 2 out]
          n131 = call "ballTargetOriented.vi"("Target"=w338, "Ball"=w332) -> ("Orientation"=w383:dbl)  [unwired: 7 in, 2 out]
          n132 = Subtract(x=w362, y=w361) -> (x-y=w360:dbl)
          n133 = Subtract(x=w383, y=w382) -> (x-y=w372:dbl)
          n134 = expression code="(x/pi)*180.0" "radians to degrees"(w372) -> (→"difAngleRobotBall 3":dbl)
          n135 = Less Or Equal?(x=w385, y=w394) -> (x <= y?=w393:bool)
          n136 = call-poly <vilib>:"Wrap Angle.vi"("angle in"=w372) -> ("angle out"=w384:dbl)  [unwired: 9 in, 1 out]
          n137 = expression code="(x/180.0)*pi" "degrees to radians"(w376) -> (w377:dbl)
          n138 = local read "pass?"() -> (w326:bool)
          n139 = Absolute Value(x=w384) -> (abs(x)=w375:dbl)
          n140 = expression code="(x/pi)*180.0" "radians to degrees"(w375) -> (→"difAngleRobotBall 4":dbl)
          n141 = Greater Or Equal?(x=w375, y=w377) -> (x >= y?=w381:bool)
          n142 = call "KickForce.vi"("KickToSkill in"=w387, "force++"=w388, "Robot"=w330, "Game"=w331, "Distance to target"=w391, "Enviroment"=w367, "kickForce"=w389, "chipKick ?"=w327, "weakKick?"=FALSE, "shootState?"=w328, "use criteria?"=w329, "pass?"=w326) -> ("kick_x Force out"=w324:dbl, "kick_z Force out"=w323:dbl)  [unwired: 4 in, 2 out]
          n143 = Greater Or Equal?(x=w385, y=w366) -> (x >= y?=w386:bool)
          n144 = Or(x=w386, y=w381) -> (x .or. y?=w380:bool)
          n145 = Select(t=robotKickToStates."walk", s=w380, f=w365) -> (s? t:f=w378:T1)
          n146 = property class="Ball"(reference=w332) -> ("position(x,y)"=w337:dbl[])  [unwired: 1 in, 2 out]
          n147 = call "dribbler.vi"("Parameters.lvclass"=w369, "Ball"=w332, "Robot"=w330, "Utilities in"=w368) -> ("Dribbler?"=w370:bool)  [unwired: 5 in, 2 out]
          n148 = call-dynamic "goBallTargetDirection.vi"("NewParameters"=w364, "Target"=w338, "state"=w365, "BallRef"=w332, "Robot"=w330, "Utilities in"=w368) -> ("dest_y"=w357:dbl, "dest_x"=w358:dbl)  [unwired: 2 in, 2 out]
          n149 = property class="Robot"(reference=w330) -> (reference out=w346:refnum<class "Robot.lvclass">, "position(x,y)"=w356:dbl[])  [unwired: 1 in, 1 out]
          n150 = Greater?(x=w360, y=3.0) -> (0:w344:bool)
          n151 = Build Array(w358, w357) -> (w350:dbl[])
          n152 = Subtract(x=w337, y=w356) -> (x-y=w354:dbl[])
          n153 = call "Module.vi"("2D vector"=w354) -> ("Modulo"=w355:dbl)  [unwired: 8 in, 2 out]
          n154 = Divide(x=w354, y=w355) -> (x/y=w353:dbl[])
          n155 = feedback #4(w342) -> (w341:dbl)
          n156 = Add(x=w342, y=w341) -> (x+y=w340:dbl)
          n157 = Select(t=w342, s=w343, f=w341) -> (s? t:f=w339:dbl)
          n158 = Select(t=w340, s=w344, f=w339) -> (s? t:f=w345:dbl)
          n159 = Multiply(x=w353, y=w345) -> (x*y=w352:dbl[])
          n160 = Add(x=w350, y=w352) -> (x+y=w351:dbl[])
          n161 = feedback-in #4(w345) -> ()
          n162 = Subtract(x=w338, y=w337) -> (x-y=w336:dbl[])
          n163 = Index Array(array=w336) -> (element #1=w335:dbl, element #2=w334:dbl)  [unwired: 2 in]
          n164 = Select(t=w351, s=w344, f=w350) -> (s? t:f=w349:dbl[])
          n165 = Inverse Tangent (2 Input)(1:w335, 2:w334) -> (0:w333:dbl)
          n166 = Index Array(array=w349) -> (element #1=w348:dbl, element #2=w347:dbl)  [unwired: 2 in]
          n167 = property class="Robot"(reference=w346, "dest_x"=w348, "dest_y"=w347, "dribble"=w370, "dest_orientation"=w333) -> (reference out=w371:refnum<class "Robot.lvclass">)  [unwired: 1 in, 1 out]
          n168 = case shown="True" w393 {
            tunnel: w371 -> [w395 w399]
            tunnel: [w395 w398] -> w392
            tunnel: w324 -> [_ w397]
            tunnel: w323 -> [_ w396]
            frame False {
            }
            frame True {
              n169 = property class="Robot"(reference=w399, "kick_x"=w397, "kick_z"=w396) -> (reference out=w398:refnum<class "Robot.lvclass">)  [unwired: 1 in, 1 out]
            }
          }
        }
      }
      n170 = call "dribbler.vi"("Parameters.lvclass"=w51, "Ball"=w34, "Robot"=w50, "Utilities in"=w46) -> ("Dribbler?"=w52:bool)  [unwired: 5 in, 2 out]
      n171 = property class="Robot"(reference=w50, "dest_x_kick"=w56, "dest_y_kick"=w55, "dribble"=w52, "robotKickState"=w25) -> (reference out=w57:refnum<class "Robot.lvclass">)  [unwired: 1 in, 1 out]
    }
    frame Error {
    }
  }
  "error out" <- w12
  "KickToSkill out" <- w10
  "Robot out" <- w8
  "State out" <- w2
  n172 = disable-structure shown="Disabled" {
    disable-tunnel: "firstCall?" -> [w404 _]
    frame Disabled {
      n173 = call "firstCallTest.vi"("firstCall"=w404) -> ("firstCallArray"=→"firstCallArray":bool[])  [unwired: 7 in, 3 out]
    }
    frame Enabled {
    }
  }
